vi "MainGui-StatusTableUpdate.vi"(8 "error in (no error)":errorcluster, 10 "TestValueResult":T1) -> (0 "error out":errorcluster)   [LabVIEW 2016]
uses:
  Database/Database.Gui.ctl
  Database/Database.Gui.SingleTestValue.ctl
  MainGui.Action.ctl
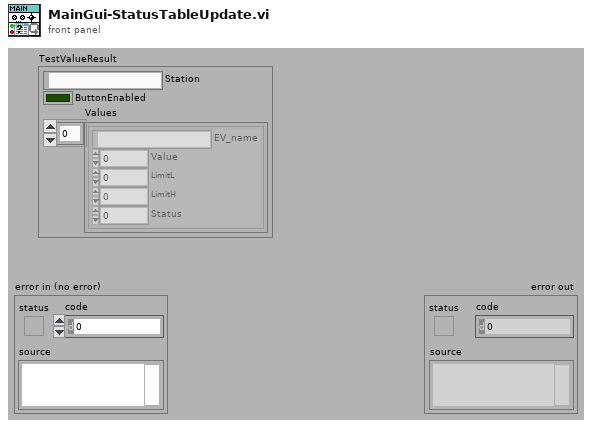
[diagram p1: front panel]
types:
  T1 = typedef "Database.Gui.ctl" = cluster{"Station":string, "ButtonEnabled":bool, "Values":T2[]}
  T2 = typedef "Database.Gui.SingleTestValue.ctl" = cluster{"EV_name":string, "Value":dbl, "LimitL":dbl, "LimitH":dbl, "Status":u8}
  T3 = typedef "MainGui.Action.ctl" = enum32{"idle", "constructor", "destructor", "--- MainGui ---", "Gui.Resize", "Gui.Translate", "Error.Update", "Error.Confirm", "TopBar.Update", "Buttons.Update", "StatusMsg.Update", "StatusTable.Update", "LogsTable.Update", "ProductList.Update", "ProductTable.Update", "SetupVariantTable.Update"}
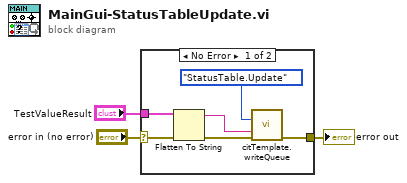
[diagram p0: block diagram]
diagram:
  n1 = case shown="No Error" "error in (no error)" {
    selector: "error in (no error)" -> [w6 w10]
    tunnel: [w9 w10] -> w2
    tunnel: "TestValueResult" -> [w7 _]
    frame No Error {
      n2 = Flatten To String(anything=w7, error in (no error)=w6) -> (data string=w4:string, error out=w5:errorcluster)  [unwired: 2 in, 1 out]
      n3 = call "citTemplate.writeQueue.vi"("event in (if not connected:all statemachine with data event)"=MainGui.Action."StatusTable.Update" ("Action"), "data in"=w4, "error in (no error)"=w5) -> ("error out"=w9:errorcluster)  [unwired: 12 in]
    }
    frame Error {
    }
  }
  "error out" <- w2
